vi "cha desc vector constructor.vi"(11 "init_cha_desc_vec":T1[](array[typedef])) -> (3 "ad_scan_cha_desc_vec":T2[](array[typedef]))   [LabVIEW 2021, in "libad4.lvlib"]
doc: "Helper function to aid in the construction of an ad_scan_cha_desc cluster/struct vector."
uses:
  <userlib>/libad4/libad4.lvlib
  <userlib>/libad4/controls/ad scan cha desc.ctl
  <userlib>/libad4/controls/init scan cha desc.ctl
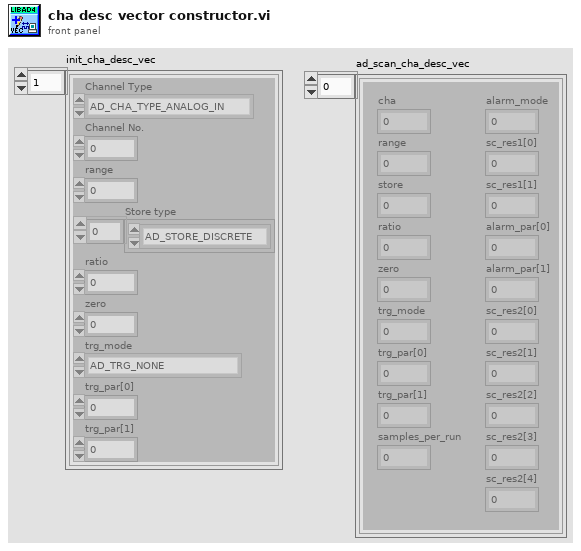
[diagram p1: front panel]
types:
  T1 = typedef "libad4.lvlib/init scan cha desc.ctl" = cluster{"Channel Type":enum16{"AD_CHA_TYPE_ANALOG_IN", "AD_CHA_TYPE_ANALOG_OUT", "AD_CHA_TYPE_DIGITAL_IO"}, "Channel No.":i32, "range":i32, "Store type":enum16{"AD_STORE_DISCRETE", "AD_STORE_AVERAGE", "AD_STORE_MIN", "AD_STORE_MAX", "AD_STORE_RMS"}[], "ratio":i32, "zero":u32, "trg_mode":enum16{"AD_TRG_NONE", "AD_TRG_POSITIVE", "AD_TRG_NEGATIVE", "AD_TRG_INSIDE", "AD_TRG_OUTSIDE", "AD_TRG_NEVER"}, "trg_par[0]":u32, "trg_par[1]":u32}
  T2 = typedef "libad4.lvlib/ad scan cha desc.ctl" = cluster{"cha":i32, "range":i32, "store":i32, "ratio":i32, "zero":u32, "trg_mode":u8, "alarm_mode":u8, "sc_res1[0]":u8, "sc_res1[1]":u8, "trg_par[0]":u32, "trg_par[1]":u32, "samples_per_run":i32, "alarm_par[0]":u32, "alarm_par[1]":u32, "sc_res2[0]":u32, "sc_res2[1]":u32, "sc_res2[2]":u32, "sc_res2[3]":u32, "sc_res2[4]":u32}
  T3 = enum16{"AD_CHA_TYPE_ANALOG_IN", "AD_CHA_TYPE_ANALOG_OUT", "AD_CHA_TYPE_DIGITAL_IO"}
  T4 = enum16{"AD_STORE_DISCRETE", "AD_STORE_AVERAGE", "AD_STORE_MIN", "AD_STORE_MAX", "AD_STORE_RMS"}[]
  T5 = enum16{"AD_TRG_NONE", "AD_TRG_POSITIVE", "AD_TRG_NEGATIVE", "AD_TRG_INSIDE", "AD_TRG_OUTSIDE", "AD_TRG_NEVER"}
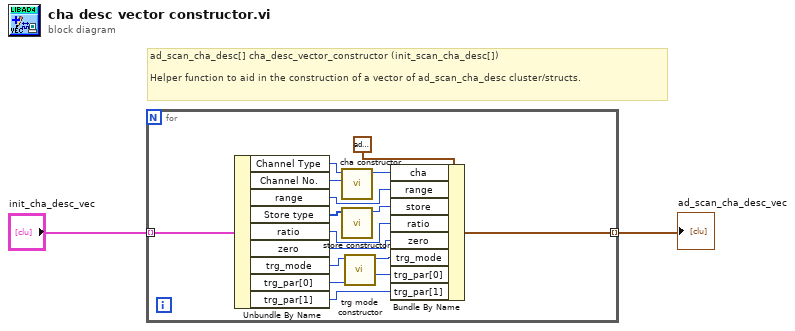
[diagram p0: block diagram]
diagram:
  # "ad_scan_cha_desc[] cha_desc_vector_constructor (init_scan_cha_desc[])\n\nHelper function to aid in the construction of a vector of ad_scan_cha_desc cluster/structs."
  n1 = for {
    tunnel: [w4] -> w2 mode=indexing
    tunnel: "init_cha_desc_vec" -> [w3] mode=indexing
    n2 = Unbundle By Name(w3) -> ("Channel Type"=w14:T3, "Channel No."=w13:i32, "range"=w12:i32, "Store type"=w11:T4, "ratio"=w10:i32, "zero"=w9:u32, "trg_mode"=w7:T5, "trg_par[0]"=w6:u32, "trg_par[1]"=w5:u32)
    n3 = call <userlib>:"cha constructor.vi"("Channel No."=w13, "Channel Type"=w14) -> ("Channel Number"=w16:i32)  [unwired: 9 in]
    n4 = call <userlib>:"store constructor.vi"("Store type"=w11) -> ("Store ID"=w15:i32)  [unwired: 10 in]
    n5 = call <userlib>:"trg mode constructor.vi"("trg_mode"=w7) -> ("trg_mode out"=w8:u8)  [unwired: 10 in]
    n6 = Bundle By Name(cluster=T2 {"cha"=0, "range"=0, "store"=0, "ratio"=0, "zero"=0, "trg_mode"=0, "alarm_mode"=0, "sc_res1[0]"=0, "sc_res1[1]"=0, "trg_par[0]"=0, "trg_par[1]"=0, "samples_per_run"=0, "alarm_par[0]"=0, "alarm_par[1]"=0, "sc_res2[0]"=0, "sc_res2[1]"=0, "sc_res2[2]"=0, "sc_res2[3]"=0, "sc_res2[4]"=0} ("ad_scan_cha_desc"), "cha"=w16, "range"=w12, "store"=w15, "ratio"=w10, "zero"=w9, "trg_mode"=w8, "trg_par[0]"=w6, "trg_par[1]"=w5) -> (w4:T2)
  }
  "ad_scan_cha_desc_vec" <- w2
